vi "Phasor Subtract Baseline from Array [SGL].vi"(0 "X Array":sgl[](array[numeric]), 1 "Method (Min)":T1=enum."Min", 2 "Gate Duration":dbl[unit]=nan, 3 "Laser Period":dbl[unit]=nan, 5 "Y Array":sgl[](array[numeric]), 7 "Max X":sgl=nan, 9 "Min X":sgl=nan, 11 "Error In":errorcluster, 12 "Background Constant":dbl) -> (4 "Bkgd-subtracted Y Array":sgl[](array[numeric]), 6 "Background/Gate":sgl, 8 "Lifetime":sgl[unit]=nan, 10 "Bkgd-subtracted Intensity (theo)":sgl, 14 "Message":string, 15 "Error Out":errorcluster)   [LabVIEW 2021, in "Phasor.lvlib"]
uses:
  Phasor.lvlib
  AlliGator/AlliGator Baseline Subtraction Method.ctl
  <vilib>/Utility/error.llb/Error Cluster From Error Code.vi
  <vilib>/ErrorRing/Error Ring.xnode
  Comparison/Comparison.lvlib
  AlliGator/AlliGator Decay Preprocessing.lvlib
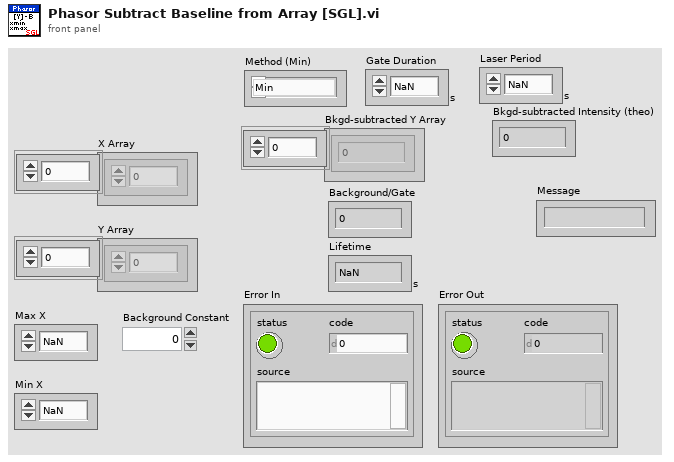
[diagram p1: front panel]
types:
  T1 = typedef "AlliGator Decay Analysis.lvlib/AlliGator Decay Preprocessing.lvlib/AlliGator Baseline Subtraction Method.ctl" = enum16{"Mean", "Min", "Square Gated Single-Exponential", "File", "Constant"}
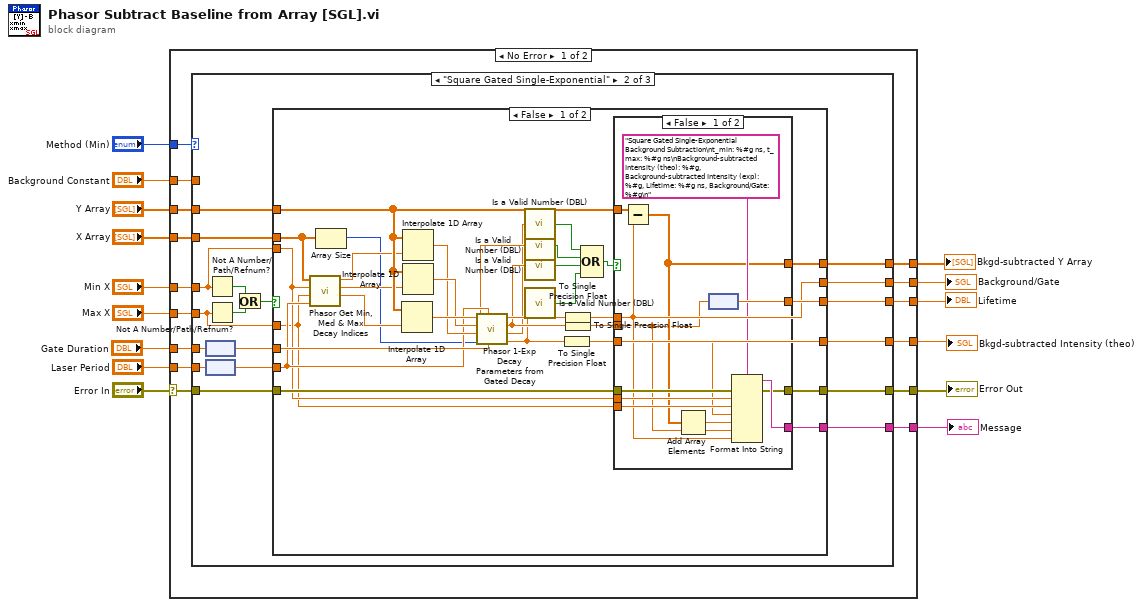
[diagram p0: block diagram]
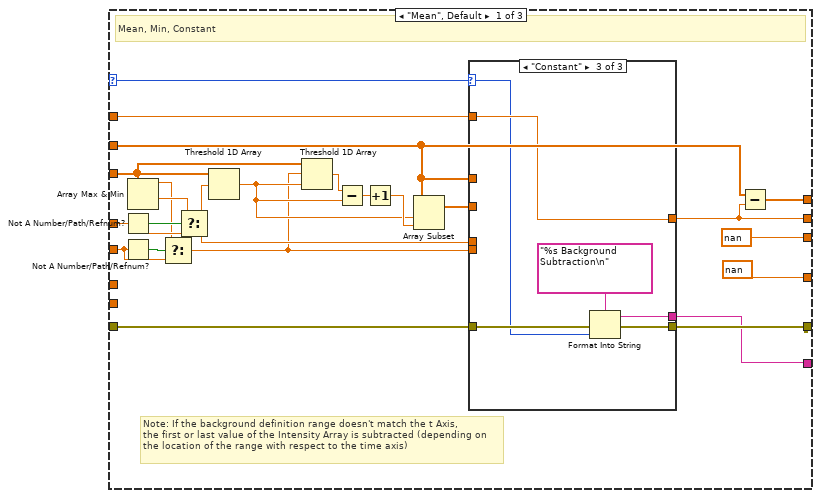
[diagram p2: hidden frame]
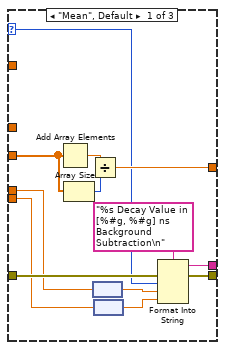
[diagram p3: hidden frame]
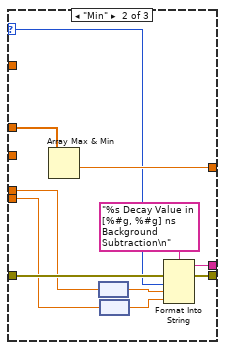
[diagram p4: hidden frame]
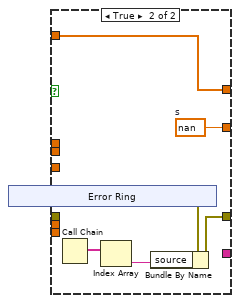
[diagram p5: hidden frame]
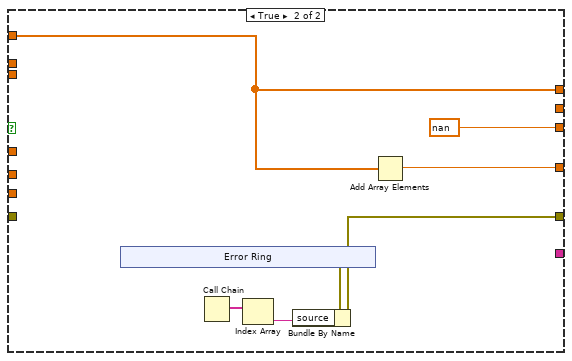
[diagram p6: hidden frame]
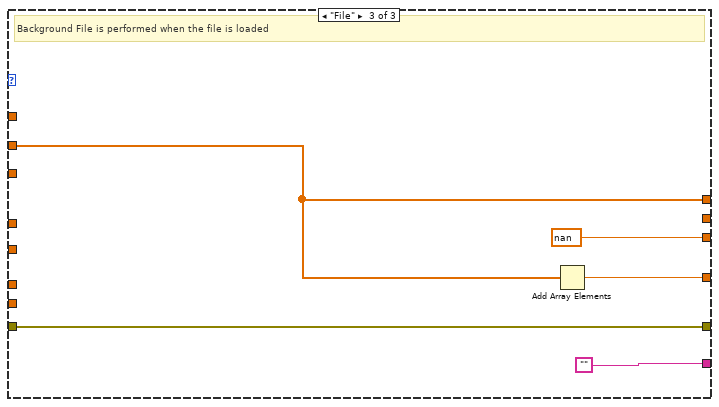
[diagram p7: hidden frame]
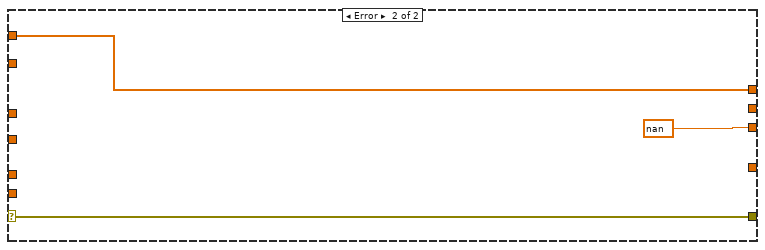
[diagram p8: hidden frame]
diagram:
  n1 = case shown="No Error" "Error In" {
    selector: "Error In" -> [w20 w174]
    tunnel: "Min X" -> [w30 _]
    tunnel: "Max X" -> [w29 _]
    tunnel: [w28 w172] -> w13
    tunnel: "X Array" -> [w27 _]
    tunnel: [w26 _] -> w11
    tunnel: "Y Array" -> [w25 w172]
    tunnel: "Method (Min)" -> [w24 _]
    tunnel: "Gate Duration" -> [w23 _]
    tunnel: "Laser Period" -> [w22 _]
    tunnel: [w21 sgl[unit] nan ("B")] -> w6
    tunnel: [w19 w174] -> w4
    tunnel: [w18 _] -> w3
    tunnel: [w17 _] -> w2
    tunnel: "Background Constant" -> [w16 _]
    frame No Error {
      n2 = case shown="\"Square Gated Single-Exponential\"" w24 {
        selector: w24 -> [w39 _ _]
        tunnel: w27 -> [w47 w91 _]
        tunnel: [w38 w94 w168] -> w28
        tunnel: [w41 w102 _] -> w26
        tunnel: w25 -> [w40 w95 w168]
        tunnel: w29 -> [w44 w89 _]
        tunnel: w30 -> [w46 w92 _]
        tunnel: w23 -> [_ w100 _]
        tunnel: w22 -> [_ w88 _]
        tunnel: [sgl[unit] nan ("B") w101 sgl[unit] nan ("B")] -> w21
        tunnel: w20 -> [w35 w93 w170]
        tunnel: [w34 w90 w170] -> w19
        tunnel: [w31 w87 ""] -> w18
        tunnel: [sgl nan ("I") w86 w167] -> w17
        tunnel: w16 -> [w36 _ _]
        frame "Mean", Default {
          # "Note: If the background definition range doesn't match the t Axis,\nthe first or last value of the Intensity Array is subtracted (depending on the location of the range with respect to the time axis)"
          # "Mean, Min, Constant"
          n3 = Not A Number/Path/Refnum?(number/path/refnum=w46) -> (NaN/Path/Refnum?=w49:bool)
          n4 = Not A Number/Path/Refnum?(number/path/refnum=w44) -> (NaN/Path/Refnum?=w48:bool)
          n5 = Array Max & Min(array=w47) -> (max value=w43:sgl, min value=w45:sgl)  [unwired: 2 out]
          n6 = Select(t=w43, s=w48, f=w44) -> (s? t:f=w32:sgl)
          n7 = Select(t=w45, s=w49, f=w46) -> (s? t:f=w33:sgl)
          n8 = Threshold 1D Array(2:w33, 3:w47) -> (0:w50:sgl)  [unwired: 1 in]
          n9 = Threshold 1D Array(1:w50, 2:w32, 3:w47) -> (0:w54:sgl)
          n10 = Subtract(x=w54, y=w50) -> (x-y=w53:sgl)
          n11 = Increment(x=w53) -> (x+1=w51:sgl)
          n12 = Array Subset(array=w40, index=w50, length=w51) -> (w52:sgl[])
          n13 = case shown="\"Constant\"" w39 {
            selector: w39 -> [w56 w68 w79]
            tunnel: w52 -> [w65 _ _]
            tunnel: [w66 w78 w84] -> w41
            tunnel: w40 -> [_ w77 _]
            tunnel: w36 -> [_ _ w84]
            tunnel: w35 -> [w60 w71 w80]
            tunnel: [w59 w72 w81] -> w34
            tunnel: w33 -> [w58 w70 _]
            tunnel: w32 -> [w57 w69 _]
            tunnel: [w55 w73 w82] -> w31
            frame "Mean", Default {
              n14 = Add Array Elements(numeric array=w65) -> (sum=w67:sgl)
              n15 = Array Size(array=w65) -> (size(s)=w64:i32)
              n16 = Divide(x=w67, y=w64) -> (x/y=w66:sgl)
              n17 = node(w58) -> (w62:sgl[unit])
              n18 = node(w57) -> (w61:sgl[unit])
              n19 = Format Into String(format string="%s Decay Value in [%#g, %#g] ns Background Subtraction\n", error in=w60, w56, w62, w61) -> (resulting string=w55:string, error out=w59:errorcluster)  [unwired: 1 in]
            }
            frame "Min" {
              n20 = Array Max & Min(array=w77) -> (min value=w78:sgl)  [unwired: 3 out]
              n21 = node(w70) -> (w75:sgl[unit])
              n22 = node(w69) -> (w74:sgl[unit])
              n23 = Format Into String(format string="%s Decay Value in [%#g, %#g] ns Background Subtraction\n", error in=w71, w68, w75, w74) -> (resulting string=w73:string, error out=w72:errorcluster)  [unwired: 1 in]
            }
            frame "Constant" {
              n24 = Format Into String(format string="%s Background Subtraction\n", error in=w80, w79) -> (resulting string=w82:string, error out=w81:errorcluster)  [unwired: 1 in]
            }
          }
          n25 = Subtract(x=w40, y=w41) -> (x-y=w38:dbl[])
        }
        frame "Square Gated Single-Exponential" {
          n26 = node(w100) -> (w99:dbl)
          n27 = node(w88) -> (w85:dbl)
          n28 = Not A Number/Path/Refnum?(number/path/refnum=w92) -> (NaN/Path/Refnum?=w98:bool)
          n29 = Not A Number/Path/Refnum?(number/path/refnum=w89) -> (NaN/Path/Refnum?=w97:bool)
          n30 = Or(x=w98, y=w97) -> (x .or. y?=w96:bool)
          n31 = case shown="False" w96 {
            tunnel: [w106 _] -> w102
            tunnel: [w132 sgl[unit] nan ("B")] -> w101
            tunnel: w99 -> [w127 _]
            tunnel: w95 -> [w131 w161]
            tunnel: [w115 w161] -> w94
            tunnel: w93 -> [w120 _]
            tunnel: w92 -> [w119 _]
            tunnel: w91 -> [w117 _]
            tunnel: [w121 w156] -> w90
            tunnel: w89 -> [w118 _]
            tunnel: w85 -> [w126 _]
            tunnel: [w122 _] -> w87
            tunnel: [w104 w160] -> w86
            frame False {
              n32 = call "Phasor Get Min, Med & Max Decay Indices.vi"("Period"=w126, "Max X"=w118, "Min X"=w119, "X Array"=w117) -> ("Max X idx"=w123:dbl, "Med X idx"=w124:dbl, "Min X idx"=w125:dbl)  [unwired: 5 in]
              n33 = Array Size(array=w117) -> (size(s)=w116:i32)
              n34 = Interpolate 1D Array(1:w123, 2:w131) -> (0:w130:sgl)
              n35 = Interpolate 1D Array(1:w125, 2:w131) -> (0:w128:sgl)
              n36 = Interpolate 1D Array(1:w124, 2:w131) -> (0:w129:sgl)
              n37 = call "Phasor 1-Exp Decay Parameters from Gated Decay.vi"("Gate Width: W"=w127, "period: T"=w126, "# Gates"=w116, "Min Decay"=w128, "Mid Decay"=w129, "Max Decay"=w130) -> ("I"=w112:dbl, "x"=w103:dbl, "tau"=w113:dbl, "B"=w114:dbl)  [unwired: 2 in]
              n38 = call "Is a Valid Number (DBL).vi"("Number"=w103) -> ("Valid Number?"=w111:bool)  [unwired: 8 in]
              n39 = call "Is a Valid Number (DBL).vi"("Number"=w114) -> ("Valid Number?"=w110:bool)  [unwired: 8 in]
              n40 = call "Is a Valid Number (DBL).vi"("Number"=w113) -> ("Valid Number?"=w109:bool)  [unwired: 8 in]
              n41 = call "Is a Valid Number (DBL).vi"("Number"=w112) -> ("Valid Number?"=w108:bool)  [unwired: 8 in]
              n42 = To Single Precision Float(number=w112) -> (single precision float=w104:sgl)
              n43 = To Single Precision Float(number=w114) -> (single precision float=w106:sgl)
              n44 = To Single Precision Float(number=w113) -> (single precision float=w105:sgl)
              n45 = Compound Arithmetic op=OR(w111, w110, w109, w108) -> (w107:bool)
              n46 = case shown="False" w107 {
                tunnel: [w145 w150] -> w132
                tunnel: w131 -> [w144 w151]
                tunnel: [w143 _] -> w122
                tunnel: [w142 w148] -> w121
                tunnel: w120 -> [w141 _]
                tunnel: w119 -> [w139 _]
                tunnel: w118 -> [w138 _]
                tunnel: [w137 w151] -> w115
                tunnel: w106 -> [w135 _]
                tunnel: w105 -> [w134 _]
                tunnel: w104 -> [w133 _]
                frame False {
                  n47 = Subtract(x=w144, y=w135) -> (x-y=w137:sgl[])
                  n48 = Add Array Elements(numeric array=w137) -> (sum=w136:sgl)
                  n49 = node(w134) -> (w145:sgl[unit])
                  n50 = Format Into String(format string="Square Gated Single-Exponential Background Subtraction\nt_min: %#g ns, t_max: %#g ns\nBackground-subtracted Intensity (theo): %#g, Background-subtracted Intensity (exp): %#g, Lifetime: %#g ns, Background/Gate: %#g\n", error in=w141, w139, w138, w133, w136, w134, w135) -> (resulting string=w143:string, error out=w142:errorcluster)  [unwired: 1 in]
                }
                frame True {
                  w150 = sgl[unit] nan  # s
                  n51 = xnode "Error Ring"() -> ("error out"=w149:errorcluster)
                  n52 = Call Chain() -> (call chain=w147:string[])
                  n53 = Index Array(array=w147) -> (element=w146:string)  [unwired: 1 in]
                  n54 = Bundle By Name(cluster=w149, "source"=w146) -> (w148:errorcluster)
                }
              }
            }
            frame True {
              n55 = xnode "Error Ring"() -> ("error out"=w157:errorcluster)
              n56 = Call Chain() -> (call chain=w159:string[])
              n57 = Index Array(array=w159) -> (element=w158:string)  [unwired: 1 in]
              n58 = Bundle By Name(cluster=w157, "source"=w158) -> (w156:errorcluster)
              n59 = Add Array Elements(numeric array=w161) -> (sum=w160:sgl)
            }
          }
        }
        frame "File" {
          # "Background File is performed when the file is loaded"
          n60 = Add Array Elements(numeric array=w168) -> (sum=w167:sgl)
        }
      }
    }
    frame Error {
    }
  }
  "Bkgd-subtracted Y Array" <- w13
  "Background/Gate" <- w11
  "Error Out" <- w4
  "Lifetime" <- w6
  "Message" <- w3
  "Bkgd-subtracted Intensity (theo)" <- w2
